vi "Store Data into Selected File Globals.vi"(0 "Sequence Ref In":refnum<k7>, 5 "Variable Names":string[](array[string]), 7 "Values to Set":dbl[](array[numeric]), 11 "error in":errorcluster, 12 "lookupString":string="DIBCalibration") -> (4 "Sequence Ref Out":refnum<k7>, 15 "error out":errorcluster)   [LabVIEW 2019]
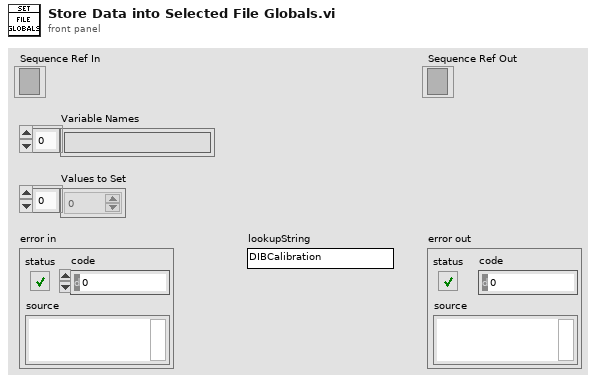
[diagram p1: front panel]
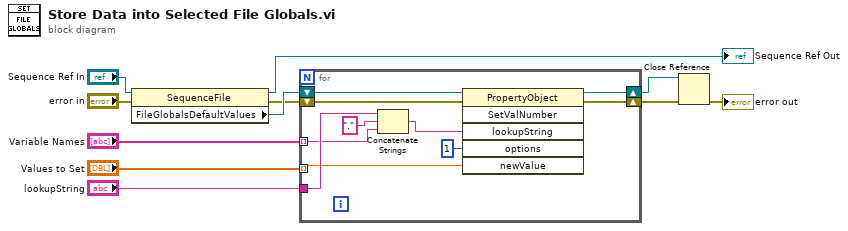
[diagram p0: block diagram]
diagram:
  n1 = property class="SequenceFile"(reference="Sequence Ref In", error in="error in") -> (reference out=→"Sequence Ref Out":refnum<k7>, error out=w6:errorcluster, "FileGlobalsDefaultValues"=w8:refnum<k7>)
  n2 = for {
    shift-right: [w21] -> w10
    shift-left: w6 -> [w15]
    shift-right: [w20] -> w3
    shift-left: w8 -> [w14]
    tunnel: "lookupString" -> [w18]
    tunnel: "Values to Set" -> [w12] mode=indexing
    tunnel: "Variable Names" -> [w13] mode=indexing
    n3 = Concatenate Strings(w18, "." ("string"), w13) -> (w16:string)
    n4 = invoke class="PropertyObject" method="SetValNumber"(reference=w14, error in=w15, "lookupString"=w16, "options"=1, "newValue"=w12) -> (reference out=w20:refnum<k7>, error out=w21:errorcluster)  [unwired: 1 in, 4 out]
  }
  n5 = Close Reference(reference=w3, error in (no error)=w10) -> (error out=→"error out":errorcluster)
